vi "getAdditionalDataFromXML.vi"(8 "error in (no error)":errorcluster, 10 "Xml":refnum<class "xmlNode.lvclass">, 11 "SingleToneRamp in":refnum<class "SingleToneRamp.lvclass">) -> (0 "error out":errorcluster, 2 "Xml out":refnum<class "xmlNode.lvclass">, 3 "SingleToneRamp out":refnum<class "SingleToneRamp.lvclass">)   [LabVIEW 2011, in "Tools.lvlib" / "Scripting.lvlib" / "SingleToneRamp.lvclass"]
uses:
  SingleToneRamp.lvclass
  xmlNode/xmlNode.lvclass
  SingleToneRamp.lvclass/SingleToneRamp.ctl
  SingleTone.lvclass
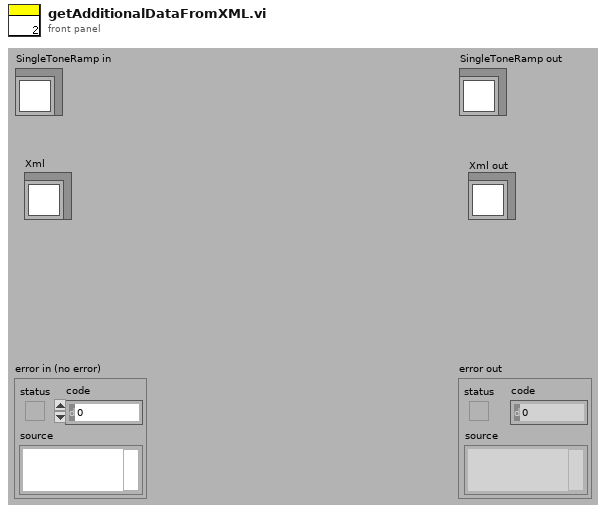
[diagram p1: front panel]
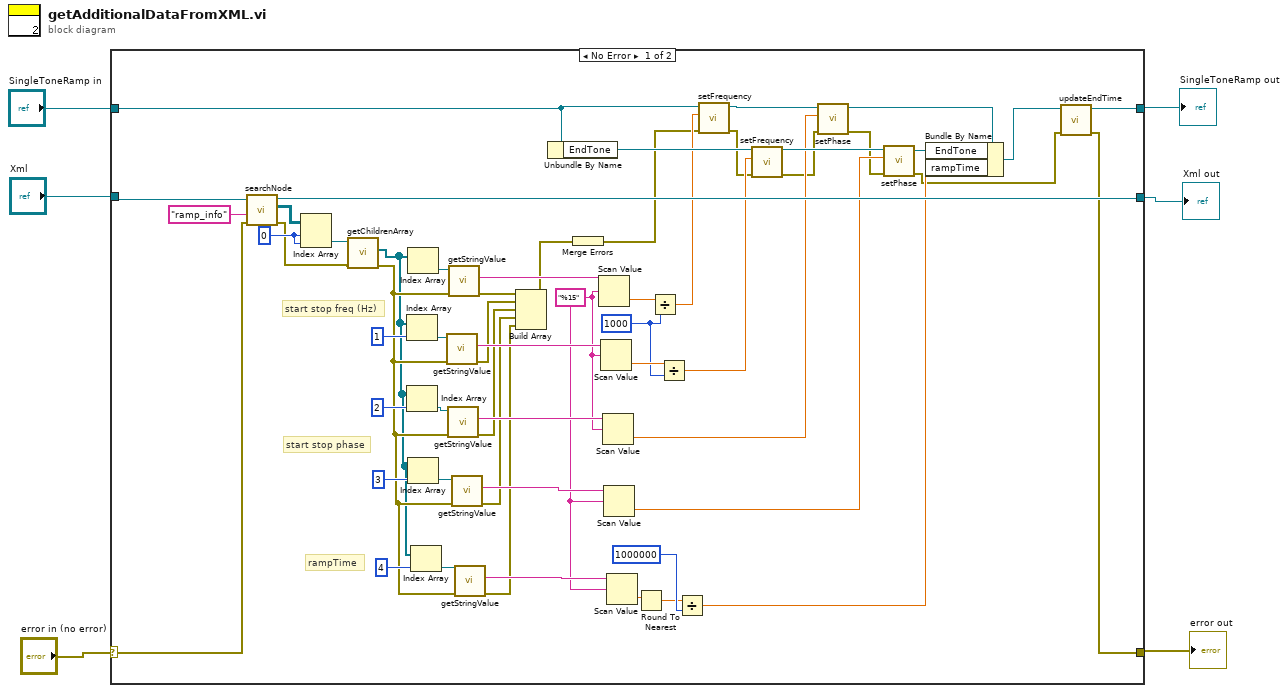
[diagram p0: block diagram]
diagram:
  n1 = case shown="No Error" "error in (no error)" {
    selector: "error in (no error)" -> [w16 w64]
    tunnel: [w15 w64] -> w5
    tunnel: [w18 w63] -> w3
    tunnel: "SingleToneRamp in" -> [w33 w63]
    tunnel: "Xml" -> [w48 _]
    tunnel: [w47 _] -> w1
    frame No Error {
      w45 = 1000
      w36 = "%15"
      w60 = 0
      # "rampTime"
      # "start stop freq (Hz)"
      # "start stop phase"
      n2 = call-dynamic "searchNode.vi"("error in (no error)"=w16, "searchElementName"="ramp_info", "xmlNode in"=w48) -> ("error out"=w58:errorcluster, "arrayXmlNodes"=w61:refnum<class "xmlNode.lvclass">[][], "xmlNode out"=w47:refnum<class "xmlNode.lvclass">)  [unwired: 6 in]
      n3 = Index Array(array=w61, index (row)=w60, index (col)=w60) -> (element=w59:refnum<class "xmlNode.lvclass">)
      n4 = call-dynamic "getChildrenArray.vi"("error in (no error)"=w58, "xmlNode.lvclass in"=w59) -> ("error out"=w38:errorcluster, "Children"=w37:refnum<class "xmlNode.lvclass">[])  [unwired: 7 in, 1 out]
      n5 = Index Array(array=w37, index=1) -> (element=w56:refnum<class "xmlNode.lvclass">)
      n6 = Index Array(array=w37, index=2) -> (element=w54:refnum<class "xmlNode.lvclass">)
      n7 = Index Array(array=w37) -> (element=w57:refnum<class "xmlNode.lvclass">)  [unwired: 1 in]
      n8 = Index Array(array=w37, index=3) -> (element=w42:refnum<class "xmlNode.lvclass">)
      n9 = Index Array(array=w37, index=4) -> (element=w39:refnum<class "xmlNode.lvclass">)
      n10 = call-dynamic "getStringValue.vi"("error in (no error)"=w38, "xmlNode.lvclass in"=w56) -> ("error out"=w13:errorcluster, "stringValue"=w51:string)  [unwired: 7 in, 1 out]
      n11 = call-dynamic "getStringValue.vi"("error in (no error)"=w38, "xmlNode.lvclass in"=w54) -> ("error out"=w12:errorcluster, "stringValue"=w49:string)  [unwired: 7 in, 1 out]
      n12 = call-dynamic "getStringValue.vi"("error in (no error)"=w38, "xmlNode.lvclass in"=w57) -> ("error out"=w14:errorcluster, "stringValue"=w52:string)  [unwired: 7 in, 1 out]
      n13 = call-dynamic "getStringValue.vi"("error in (no error)"=w38, "xmlNode.lvclass in"=w42) -> ("error out"=w11:errorcluster, "stringValue"=w43:string)  [unwired: 7 in, 1 out]
      n14 = call-dynamic "getStringValue.vi"("error in (no error)"=w38, "xmlNode.lvclass in"=w39) -> ("error out"=w10:errorcluster, "stringValue"=w40:string)  [unwired: 7 in, 1 out]
      n15 = Build Array(w14, w13, w12, w11, w10) -> (w9:errorcluster[])
      n16 = Unbundle By Name(w33) -> ("EndTone"=w32:refnum<class "SingleTone.lvclass">)
      n17 = Merge Errors(w9) -> (w8:errorcluster)
      n18 = Scan Value(string=w52, format string=w36) -> (value=w50:dbl)  [unwired: 1 in, 1 out]
      n19 = Scan Value(string=w51, format string=w36) -> (value=w46:dbl)  [unwired: 1 in, 1 out]
      n20 = Scan Value(string=w49, format string=w36) -> (value=w26:dbl)  [unwired: 1 in, 1 out]
      n21 = Scan Value(string=w43, format string=w36) -> (value=w25:dbl)  [unwired: 1 in, 1 out]
      n22 = Scan Value(string=w40, format string=w36) -> (value=w35:dbl)  [unwired: 1 in, 1 out]
      n23 = Round To Nearest(number=w35) -> (nearest integer value=w7:dbl)
      n24 = Divide(x=w50, y=w45) -> (x/y=w31:dbl)
      n25 = Divide(x=w46, y=w45) -> (x/y=w30:dbl)
      n26 = Divide(x=w7, y=1000000) -> (x/y=w20:dbl)
      n27 = call "setFrequency.vi"("error in (no error)"=w8, "frequency"=w31, "SingleTone.lvclass in"=w33) -> ("error out"=w29:errorcluster, "SingleTone.lvclass out"=w28:refnum<class "SingleToneRamp.lvclass">)  [unwired: 7 in]
      n28 = call "setFrequency.vi"("error in (no error)"=w29, "frequency"=w30, "SingleTone.lvclass in"=w32) -> ("error out"=w24:errorcluster, "SingleTone.lvclass out"=w27:refnum<class "SingleTone.lvclass">)  [unwired: 7 in]
      n29 = call "setPhase.vi"("error in (no error)"=w24, "phase"=w26, "SingleTone.lvclass in"=w28) -> ("error out"=w23:errorcluster, "SingleTone.lvclass out"=w22:refnum<class "SingleToneRamp.lvclass">)  [unwired: 7 in]
      n30 = call "setPhase.vi"("error in (no error)"=w23, "phase"=w25, "SingleTone.lvclass in"=w27) -> ("error out"=w17:errorcluster, "SingleTone.lvclass out"=w21:refnum<class "SingleTone.lvclass">)  [unwired: 7 in]
      n31 = Bundle By Name(cluster=w22, "EndTone"=w21, "rampTime"=w20) -> (w19:refnum<class "SingleToneRamp.lvclass">)
      n32 = call-dynamic "updateEndTime.vi"("error in (no error)"=w17, "SingleToneRamp in"=w19) -> ("error out"=w15:errorcluster, "SingleToneRamp out"=w18:refnum<class "SingleToneRamp.lvclass">)  [unwired: 8 in]
    }
    frame Error {
    }
  }
  "error out" <- w5
  "SingleToneRamp out" <- w3
  "Xml out" <- w1
